vi "Delete_every_nth_element.vi"(1 "n":i32=20, 2 "System Monitor Variables":T1={"Time"=[], "LI1CH1"=[], "LI1CH2"=[], "LI2CH1"=[], "LI2CH2"=[], "LI3CH1"=[], "LI3CH2"=[], "Field"=[], "N_Level"=[], "H_Level"=[], "Heat_370"=[], "Sorb_Heat"=[], "Still_Heat"=[], "Capacity"=[], "Loss"=[], "Magnet_Temperature"=[], "Lam_Pressure"=[], "Lam_NValve"=[], "370-T1"=[], "370-T2"=[], "370-T3"=[], "370-T4"=[], "370-T5"=[], "370-R1"=[], "370-R2"=[], "370-R3"=[], "370-R4"=[], "370-R5"=[], "372-T1"=[], "372-T2"=[], "372-T3"=[], "372-T4"=[], "372-T5"=[], "372-T6"=[], "372-R1"=[], "372-R2"=[], "372-R3"=[], "372-R4"=[], "372-R5"=[], "372-R6"=[], "Nada"=[nan], "K2440_Res"=[], "K2440_Current"=[], "VTI_Heater"=[], "VTI_NValve"=[], "LS340_Heater"=[], "K6221_Amplitude"=[], "K6221_Frequency"=[], "Cond_Pressure"=[], "Still_Pressure"=[], "FP_Out_Pressure"=[], "Dump_Pressure"=[], "V1"=[], "V2"=[], "V4"=[], "V5"=[], "V9"=[], "Forepump"=[], "Compressor"=[], "K6221_Offset"=[], "BoxTemp"=[], "By"=[], "Bz"=[], "Phi"=[], "heater-recond (%)"=[], "Dewar Pressure "=[], "JT-SP-Control"=[], "350 T1"=[], "350 T2"=[], "350 T3"=[], "350 T4"=[], "350 R1"=[], "350 R2"=[], "350 R3"=[], "350 R4"=[], "Angle"=[], "VTI CH1"=[], "VTI CH2"=[], "VTI CH3"=[]}) -> (0 "System Monitor Variables 2":T1={"Time"=[], "LI1CH1"=[], "LI1CH2"=[], "LI2CH1"=[], "LI2CH2"=[], "LI3CH1"=[], "LI3CH2"=[], "Field"=[], "N_Level"=[], "H_Level"=[], "Heat_370"=[], "Sorb_Heat"=[], "Still_Heat"=[], "Capacity"=[], "Loss"=[], "Magnet_Temperature"=[], "Lam_Pressure"=[], "Lam_NValve"=[], "370-T1"=[], "370-T2"=[], "370-T3"=[], "370-T4"=[], "370-T5"=[], "370-R1"=[], "370-R2"=[], "370-R3"=[], "370-R4"=[], "370-R5"=[], "372-T1"=[], "372-T2"=[], "372-T3"=[], "372-T4"=[], "372-T5"=[], "372-T6"=[], "372-R1"=[], "372-R2"=[], "372-R3"=[], "372-R4"=[], "372-R5"=[], "372-R6"=[], "Nada"=[nan], "K2440_Res"=[], "K2440_Current"=[], "VTI_Heater"=[], "VTI_NValve"=[], "LS340_Heater"=[], "K6221_Amplitude"=[], "K6221_Frequency"=[], "Cond_Pressure"=[], "Still_Pressure"=[], "FP_Out_Pressure"=[], "Dump_Pressure"=[], "V1"=[], "V2"=[], "V4"=[], "V5"=[], "V9"=[], "Forepump"=[], "Compressor"=[], "K6221_Offset"=[], "BoxTemp"=[], "By"=[], "Bz"=[], "Phi"=[], "heater-recond (%)"=[], "Dewar Pressure "=[], "JT-SP-Control"=[], "350 T1"=[], "350 T2"=[], "350 T3"=[], "350 T4"=[], "350 R1"=[], "350 R2"=[], "350 R3"=[], "350 R4"=[], "Angle"=[], "VTI CH1"=[], "VTI CH2"=[], "VTI CH3"=[]})   [LabVIEW 2016]
uses:
  Global/Global Variables/System Monitor Cluster.ctl
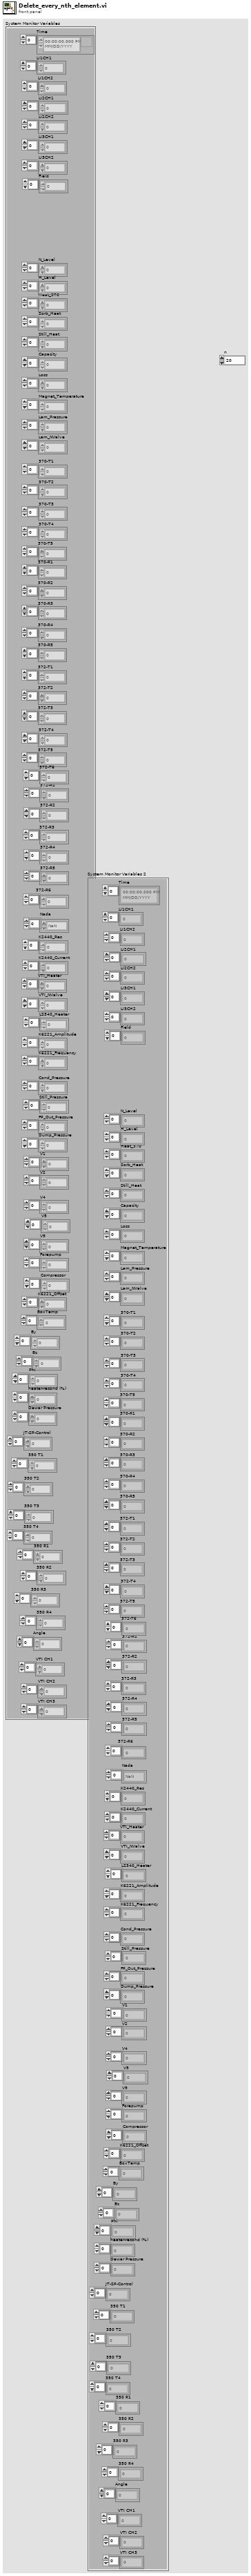
[diagram p1: front panel]
types:
  T1 = typedef "System Monitor Cluster.ctl" = cluster{"Time":timestamp[], "LI1CH1":dbl[], "LI1CH2":dbl[], "LI2CH1":dbl[], "LI2CH2":dbl[], "LI3CH1":dbl[], "LI3CH2":dbl[], "Field":dbl[], "N_Level":dbl[], "H_Level":dbl[], "Heat_370":dbl[], "Sorb_Heat":dbl[], "Still_Heat":dbl[], "Capacity":dbl[], "Loss":dbl[], "Magnet_Temperature":dbl[], "Lam_Pressure":dbl[], "Lam_NValve":dbl[], "370-T1":dbl[], "370-T2":dbl[], "370-T3":dbl[], "370-T4":dbl[], "370-T5":dbl[], "370-R1":dbl[], "370-R2":dbl[], "370-R3":dbl[], "370-R4":dbl[], "370-R5":dbl[], "372-T1":dbl[], "372-T2":dbl[], "372-T3":dbl[], "372-T4":dbl[], "372-T5":dbl[], "372-T6":dbl[], "372-R1":dbl[], "372-R2":dbl[], "372-R3":dbl[], "372-R4":dbl[], "372-R5":dbl[], "372-R6":dbl[], "Nada":dbl[], "K2440_Res":dbl[], "K2440_Current":dbl[], "VTI_Heater":dbl[], "VTI_NValve":dbl[], "LS340_Heater":dbl[], "K6221_Amplitude":dbl[], "K6221_Frequency":dbl[], "Cond_Pressure":dbl[], "Still_Pressure":dbl[], "FP_Out_Pressure":dbl[], "Dump_Pressure":dbl[], "V1":dbl[], "V2":dbl[], "V4":dbl[], "V5":dbl[], "V9":dbl[], "Forepump":dbl[], "Compressor":dbl[], "K6221_Offset":dbl[], "BoxTemp":dbl[], "By":dbl[], "Bz":dbl[], "Phi":dbl[], "heater-recond (%)":dbl[], "Dewar Pressure ":dbl[], "JT-SP-Control":dbl[], "350 T1":dbl[], "350 T2":dbl[], "350 T3":dbl[], "350 T4":dbl[], "350 R1":dbl[], "350 R2":dbl[], "350 R3":dbl[], "350 R4":dbl[], "Angle":dbl[], "VTI CH1":dbl[], "VTI CH2":dbl[], "VTI CH3":dbl[]}
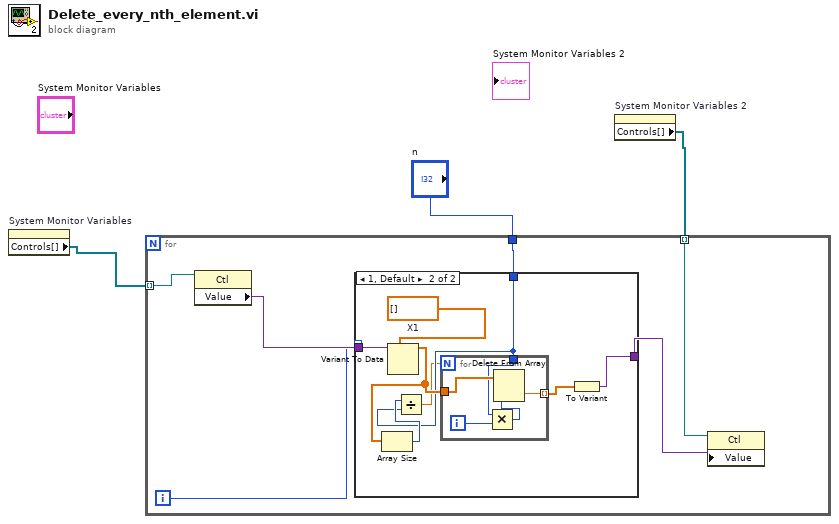
[diagram p0: block diagram]
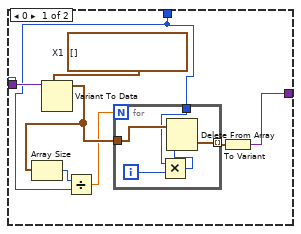
[diagram p2: hidden frame]
diagram:
  n1 = property on="System Monitor Variables" class="Clust (strict)"() -> ("Controls[]"=w2:refnum<vi>[])  [unwired: 2 in, 2 out]
  n2 = property on="System Monitor Variables 2" class="Clust (strict)"() -> ("Controls[]"=w1:refnum<vi>[])  [unwired: 2 in, 2 out]
  n3 = for {
    tunnel: w2 -> [w9] mode=indexing
    tunnel: "n" -> [w5]
    tunnel: w1 -> [w7] mode=indexing
    i -> [w6]
    n4 = property class="Ctl"(reference=w9) -> ("Value"=w8:variant)  [unwired: 1 in, 2 out]
    n5 = case shown="1, Default" w6 {
      tunnel: w8 -> [w17 w30]
      tunnel: [w15 w28] -> w4
      tunnel: w5 -> [w11 w24]
      frame 0 {
        w16 = timestamp[] []  # X1
        n6 = Variant To Data(type=w16, Variant=w17) -> (data=w13:timestamp[])  [unwired: 1 in, 1 out]
        n7 = Array Size(array=w13) -> (size(s)=w12:i32)
        n8 = Divide(x=w12, y=w11) -> (x/y=w10:dbl)
        n9 = for {
          N: w10 -> [_]
          tunnel: w13 -> [w22]
          tunnel: w11 -> [w20]
          tunnel: [w18] -> w14 mode=indexing
          i -> [w21]
          n10 = Multiply(x=w20, y=w21) -> (x*y=w19:i32)
          n11 = Delete From Array(array=w22, index=w19) -> (deleted portion=w18:timestamp)  [unwired: 1 in, 1 out]
        }
        n12 = To Variant(anything=w14) -> (Variant=w15:variant)
      }
      frame 1, Default {
        w29 = dbl[] []  # X1
        n13 = Variant To Data(type=w29, Variant=w30) -> (data=w26:dbl[])  [unwired: 1 in, 1 out]
        n14 = Array Size(array=w26) -> (size(s)=w25:i32)
        n15 = Divide(x=w25, y=w24) -> (x/y=w23:dbl)
        n16 = for {
          N: w23 -> [_]
          tunnel: w26 -> [w35]
          tunnel: w24 -> [w33]
          tunnel: [w31] -> w27 mode=indexing
          i -> [w34]
          n17 = Multiply(x=w33, y=w34) -> (x*y=w32:i32)
          n18 = Delete From Array(array=w35, index=w32) -> (deleted portion=w31:dbl)  [unwired: 1 in, 1 out]
        }
        n19 = To Variant(anything=w27) -> (Variant=w28:variant)
      }
    }
    n20 = property class="Ctl"(reference=w7, "Value"=w4) -> ()  [unwired: 1 in, 2 out]
  }
